vi "UDP Data Link - Configuration Utilities - Add Channel.vi"(5 "Channel Path Sources":string[](array[string]), 6 "Rx Channel Name":string, 7 "Channel Path Destinations":string[](array[string]), 8 "error in (no error)":errorcluster, 9 "Rx Channel Ref":T1 format="%.0x", 10 "Dependent Node Ref":T1 format="%.0x", 11 "Rx Section Ref in":T1 format="%.0x") -> (0 "error out":errorcluster, 3 "Rx Section Ref in":T1 format="%.0x")   [LabVIEW 2015, in "UDP-Custom-Device System Explorer.lvlib"]
uses:
  UDP-Custom-Device System Explorer.lvlib
  <vilib>/NI Veristand/Custom Device API/Custom Device Item Ref.ctl
  <vilib>/NI Veristand/Custom Device API/Custom Device Channel.ctl
  <vilib>/NI Veristand/Custom Device API/Custom Device Channel Type.ctl
  Shared/Constants.vi
  <vilib>/NI Veristand/Custom Device API/Set Item Property (Dependent Node Pointer).vi
  <vilib>/NI VeriStand/Custom Device API/Custom Device API.lvlib
  Shared/UDP-Custom-Device Shared.lvlib
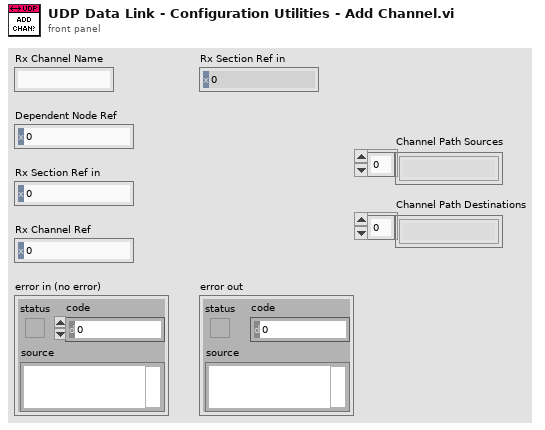
[diagram p1: front panel]
types:
  T1 = typedef "Custom Device API.lvlib/Custom Device Item Ref.ctl" = u64
  T2 = cluster{"Channel Names":string[], "Channel Paths":string[], "Dependent Node References":T1[]}
  T3 = typedef "Custom Device API.lvlib/Custom Device Channel.ctl" = cluster{"Type":T4, "Units":string, "Default Value":dbl, "Faultable":bool, "Scalable":bool}
  T4 = typedef "Custom Device API.lvlib/Custom Device Channel Type.ctl" = enum16{"Input", "Output"}
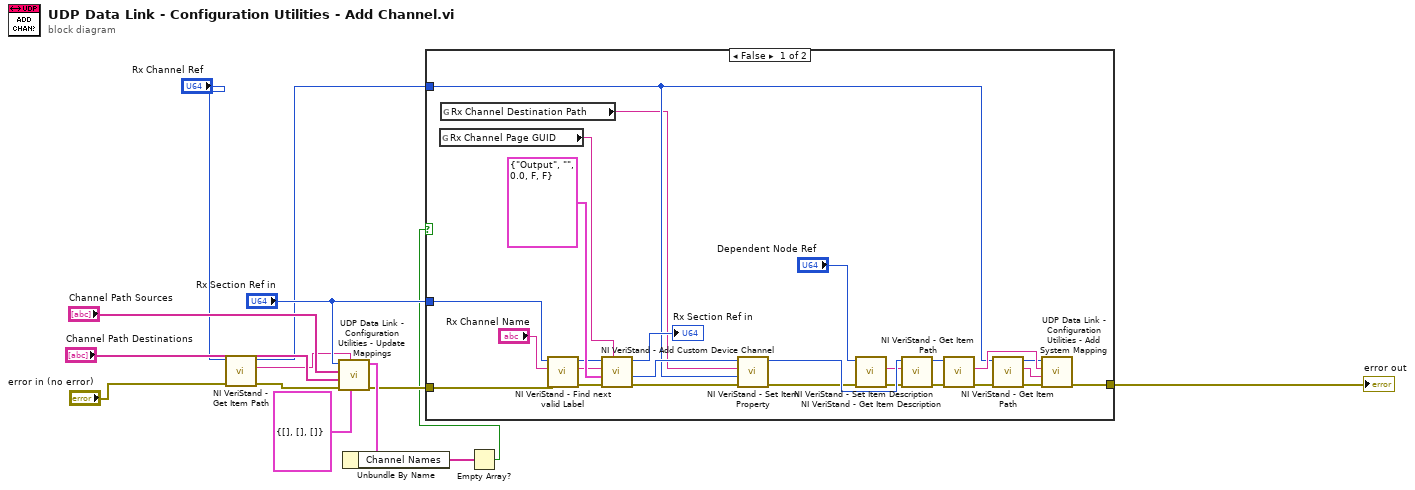
[diagram p0: block diagram]
diagram:
  n1 = call <vilib>:"NI VeriStand - Get Item Path.vi"("error in (no error)"="error in (no error)", "Item Ref in"="Rx Channel Ref") -> ("error out"=w8:errorcluster, "Path"=w7:string, "Item Ref out"=w5:T1)  [unwired: 6 in, 1 out]
  n2 = call "UDP Data Link - Configuration Utilities - Update Mappings.vi"("Channel Data in"=T2 {"Channel Names"=[], "Channel Paths"=[], "Dependent Node References"=[]}, "Channel Path"=w7, "error in (no error)"=w8, "Channel Path Destinations"="Channel Path Destinations", "Channel Path Sources"="Channel Path Sources", "Item Ref in"="Rx Section Ref in") -> ("error out"=w2:errorcluster, "Channel Data out"=w4:T2)  [unwired: 4 in]
  n3 = Unbundle By Name(w4) -> ("Channel Names"=w3:string[])
  n4 = Empty Array?(array=w3) -> (empty?=w1:bool)
  n5 = case shown="False" w1 {
    tunnel: [w33 w41] -> w14
    tunnel: "Rx Section Ref in" -> [w20 _]
    tunnel: w5 -> [w19 _]
    tunnel: w2 -> [w17 w41]
    frame False {
      n6 = global read "Constants.vi" "Rx Channel Page GUID"() -> (w16:string)
      n7 = global read "Constants.vi" "Rx Channel Destination Path"() -> (w15:string)
      n8 = call <vilib>:"NI VeriStand - Find next valid Label.vi"("error in (no error)"=w17, "Label"="Rx Channel Name", "Item Ref in"=w20) -> ("error out"=w22:errorcluster, "Label out"=w23:string, "Item Ref out"=w21:T1)  [unwired: 4 in, 2 out]
      n9 = call <vilib>:"NI VeriStand - Add Custom Device Channel.vi"("GUID (Default Channel)"=w16, "error in (no error)"=w22, "Channel"=T3 {"Type"=enum."Output", "Units"="", "Default Value"=0.0, "Faultable"=FALSE, "Scalable"=FALSE}, "Channel Name"=w23, "Parent Ref in"=w21) -> ("error out"=w29:errorcluster, "Channel Ref"=w31:T1, "Parent Ref out"=→"Rx Section Ref in":T1)  [unwired: 3 in, 1 out]
      n10 = call-poly <vilib>:"NI VeriStand - Set Item Property.vi"("error in (no error)"=w29, "Dependent Node Ref"=w19, "Property Name"=w15, "Item Ref in"=w31) -> ("error out"=w30:errorcluster, "Item Ref out"=w32:T1)  [unwired: 5 in, 1 out]
      n11 = call <vilib>:"NI VeriStand - Get Item Description.vi"("error in (no error)"=w30, "Item Ref in"="Dependent Node Ref") -> ("error out"=w26:errorcluster, "Description"=w27:string)  [unwired: 6 in, 2 out]
      n12 = call <vilib>:"NI VeriStand - Set Item Description.vi"("error in (no error)"=w26, "Description"=w27, "Item Ref in"=w32) -> ("error out"=w34:errorcluster, "Item Ref out"=w35:T1)  [unwired: 6 in, 1 out]
      n13 = call <vilib>:"NI VeriStand - Get Item Path.vi"("error in (no error)"=w34, "Item Ref in"=w35) -> ("error out"=w36:errorcluster, "Path"=w39:string)  [unwired: 6 in, 2 out]
      n14 = call <vilib>:"NI VeriStand - Get Item Path.vi"("error in (no error)"=w36, "Item Ref in"=w19) -> ("error out"=w37:errorcluster, "Path"=w40:string, "Item Ref out"=w38:T1)  [unwired: 6 in, 1 out]
      n15 = call "UDP Data Link - Configuration Utilities - Add System Mapping.vi"("error in (no error)"=w37, "Channel Path Destination"=w40, "Channel Path Source"=w39, "Item Ref in"=w38) -> ("error out"=w33:errorcluster)  [unwired: 6 in, 1 out]
    }
    frame True {
    }
  }
  "error out" <- w14
